vi "2ndStrikerNormalV2.vi"(0 "Início de pass state":bool=TRUE, 4 "Impulso de\ntime elapsed":bool=TRUE, 5 "Force Start":bool, 6 "atacando ao contrário?":bool=TRUE, 7 "AI Parameters":T1={"GotoKick"={"Dist do cone a frente"=150.0, "attacker farback"=1500.0, "Perto"=300.0, "min dist to kick"=150.0, "kick eps"=0.0, "Time to transition"=0.05}, "Attacker"={"CC chute"=0.09, "CC passe"=0.045, "Kick Force"=100.0, "ball-robot Kick"=200.0, "ball-robot Pass"=0.3, "drible\nAttk"=FALSE}, "Defender"={"D max"=1700.0, "Vel p/ robô av"=1000.0, "Kick Force"=100.0, "D atk-def"=0.0, "D farback"=0.0, "drible\ndef"=FALSE, "drible\ngoalie"=FALSE}, "Timeout"={"Field/v in x"=6.0, "Dist Robots"=300, "Dist up in y"=300}, "Pose Striker"={"dist"=200.0, "Numeric"=-4.0, "dist 2"=200.0, "drible\nstriker"=FALSE}, "Dist Stop"=300.0, "D ball out"=200, "D central gap "=150.0, "T pass"=0.0, "Force ++"=0.0, "range kick"=0.0, "Chute alto"=TRUE, "Marcador novo"=TRUE, "drible"=FALSE, "D drible"=300.0, "Versão Striker"=enum."3", "Defesa"=enum."ManMark", "Marcador"=enum."Marcar Segundo mais perigoso", "Receptor passe"=enum."2nd Striker", "Área"=enum."Quadrada"} {"D drible" format="%#_13g"; "D central gap" format="%#_13g"; "Dist Stop" format="%#_13g"; "Pose Striker"."Numeric" format="%#_13g"; "Defender"."Kick Force" format="%#_13g"; "Defender"."Vel p/ robô av" format="%#_13g"; "Attacker"."ball-robot Kick" format="%#_13g"; "Attacker"."Kick Force" format="%#_13g"; "Attacker"."CC passe" format="%#_13g"; "Attacker"."CC chute" format="%#_13g"; "GotoKick"."kick eps" format="%#_13g"; "GotoKick"."min dist to kick" format="%#_13g"; "GotoKick"."Perto" format="%#_13g"; "GotoKick"."attacker farback" format="%#_13g"; "GotoKick"."Dist do cone a frente" format="%#_13g"}, 8 "IA Input":T9={"our_robots"=[], "enemy_robots"=[], "balls"=[], "geometry"={"line_width"=0, "field_length"=0, "field_width"=0, "boundary_width"=0, "referee_width"=0, "goal_width"=0, "goal_depth"=0, "goal_wall_width"=0, "center_circle_radius"=0, "defense_radius"=0, "defense_stretch"=0, "free_kick_from_defense_dist"=0, "penalty_spot_from_field_line_dist"=0, "penalty_line_from_spot_dist"=0}, "IA Judge"={"stage"="", "command"="", "our_goalie_id"=0.0, "enemy_goalie_id"=0.0, "command enum"=enum."Halt", "Time"=enum."Azul"}, "Received Timestamp"=timestamp(0 s since 1904-01-01), "Events"={"Touch"=FALSE, "Ball out"=FALSE, "id touch"=0.0, "Ball out of \nVision"=FALSE, "Ball inside \nGoalie area"=FALSE, "Robot not responding"=FALSE, "Robots responding status"=[1.0, 1.0, 1.0, 1.0, 1.0, 1.0], "Enemy Ball \nPossession"=FALSE, "Pass State"=FALSE, "id end of pass"=0.0, "Kick"=FALSE, "Id ini Possession"=0.0, "Ball Possesion"=FALSE, "Id Possesion"=0.0, "Direct Kick"=FALSE, "2nd Strk Ativo"=FALSE}}, 9 "balls":T7[](array[typedef])=[{"x"=-2165.869384765625, "y"=510.4085693359375, "timestamp"=timestamp(2082758857.4639893 s since 1904-01-01), "Vel_x"=0.0, "Vel_y"=0.0, "Pos Bola Est"=[]}], 10 "Field Size in":T8={"line_width"=10, "field_length"=6000, "field_width"=4000, "boundary_width"=250, "referee_width"=425, "goal_width"=700, "goal_depth"=180, "goal_wall_width"=20, "center_circle_radius"=500, "defense_radius"=500, "defense_stretch"=350, "free_kick_from_defense_dist"=700, "penalty_spot_from_field_line_dist"=450, "penalty_line_from_spot_dist"=350}, 11 "Robot in":T2={"id"=5, "function"=enum."Attacker", "x"=-1842.5054931640625, "y"=520.60986328125, "orientation"=-2.7555055618286133, "v_tangent"=0.0, "v_normal"=0.0, "v_ang"=0.0, "kick_x"=0.0, "kick_z"=0.0, "dribble"=FALSE, "Timestamp"=timestamp(2082758857.4639893 s since 1904-01-01), "estimatives"={"est_v_tangent"=0.0, "est_v_normal"=0.0, "est_vx"=0.0, "est_vy"=0.0, "Pos Robot Est"=[]}, "dest_x_kick"=0.0, "dest_y_kick"=0.0, "Gap Coord"=[], "States"=enum."GoToTangent", "Path "=[], "Path  Smooth"=[], "Dest"=[]}) -> (2 "Robot out":T2={"id"=5, "function"=enum."Attacker", "x"=-1842.5054931640625, "y"=520.60986328125, "orientation"=-2.7555055618286133, "v_tangent"=-0.08361641967936218, "v_normal"=-0.20513016702014014, "v_ang"=0.24456003022714357, "kick_x"=0.0, "kick_z"=0.0, "dribble"=FALSE, "Timestamp"=timestamp(2082758857.4639893 s since 1904-01-01), "estimatives"={"est_v_tangent"=0.0, "est_v_normal"=0.0, "est_vx"=0.0, "est_vy"=0.0, "Pos Robot Est"=[]}, "dest_x_kick"=0.0, "dest_y_kick"=0.0, "Gap Coord"=[], "States"=enum."GoToTangent", "Path "=[], "Path  Smooth"=[], "Dest"=[]})   [LabVIEW 2017]
uses:
  Core/AI Robot.ctl
  Functions Enum.ctl
  AttackerStates.ctl
  Path Planning/RRT/PathDests.ctl
  Path Planning/RRT/PathDest.ctl
  Core/AI Input.ctl
  Core/AI Ball.ctl
  Core/Field Size.ctl
  Core/AI Judge.ctl
  Command Enum.ctl
  Util/Events/Events.ctl
  AI Parameters.ctl
panel:
  in  "Wait pass perpendicular?":bool=TRUE
  in  "Marcador sempre":bool
  out "size(s)":i32
  in  "IDattacker":dbl
  in  "Yattacker":dbl
  in  "Xattacker":dbl
  out "States":T4
  out "sentido":dbl
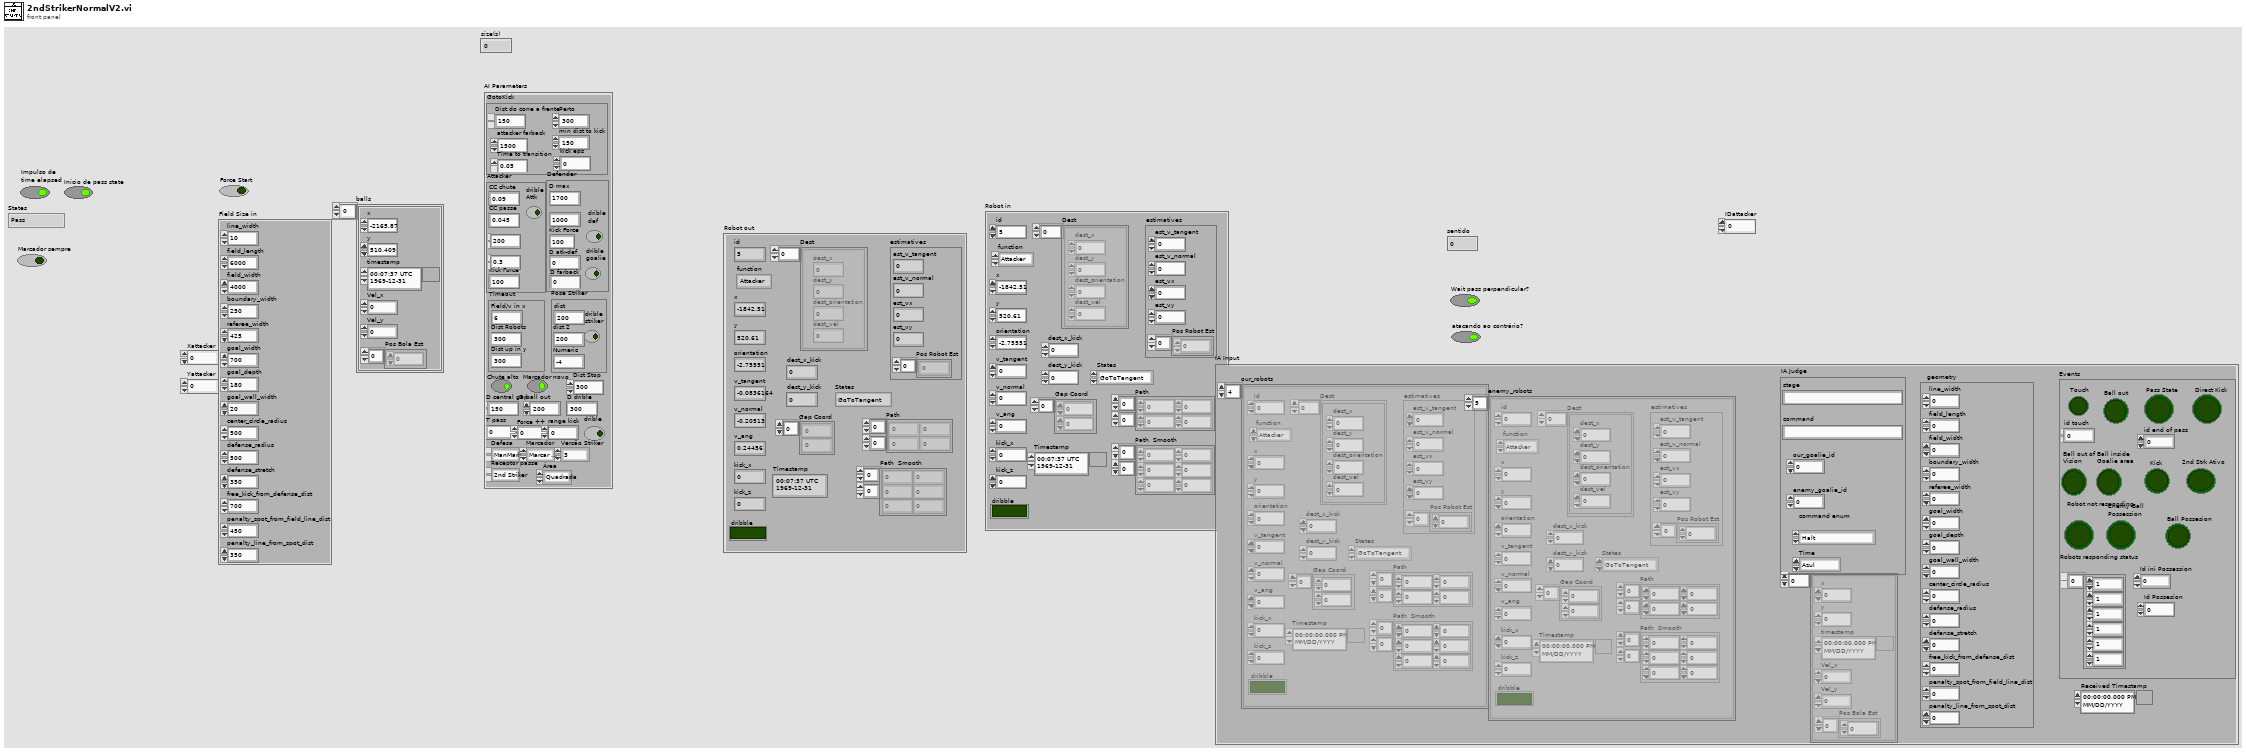
[diagram p1: front panel]
types:
  T1 = typedef "AI Parameters.ctl" = cluster{"GotoKick":cluster{"Dist do cone a frente":dbl, "attacker farback":dbl, "Perto":dbl, "min dist to kick":dbl, "kick eps":dbl, "Time to transition":dbl}, "Attacker":cluster{"CC chute":dbl, "CC passe":dbl, "Kick Force":dbl, "ball-robot Kick":dbl, "ball-robot Pass":dbl, "drible\nAttk":bool}, "Defender":cluster{"D max":dbl, "Vel p/ robô av":dbl, "Kick Force":dbl, "D atk-def":dbl, "D farback":dbl, "drible\ndef":bool, "drible\ngoalie":bool}, "Timeout":cluster{"Field/v in x":dbl, "Dist Robots":u32, "Dist up in y":u32}, "Pose Striker":cluster{"dist":dbl, "Numeric":dbl, "dist 2":dbl, "drible\nstriker":bool}, "Dist Stop":dbl, "D ball out":i32, "D central gap ":dbl, "T pass":dbl, "Force ++":dbl, "range kick":dbl, "Chute alto":bool, "Marcador novo":bool, "drible":bool, "D drible":dbl, "Versão Striker":enum16{"Auto", "3", "2", "1"}, "Defesa":enum16{"ManMark", "Barreira"}, "Marcador":enum16{"Marcar Segundo mais perigoso", "Marcar o mais perigoso"}, "Receptor passe":enum16{"Auto", "2nd Striker", "Striker"}, "Área":enum16{"Quadrada", "Circular"}}
  T2 = typedef "AI Robot.ctl" = cluster{"id":u32, "function":T3, "x":dbl, "y":dbl, "orientation":dbl, "v_tangent":dbl, "v_normal":dbl, "v_ang":dbl, "kick_x":dbl, "kick_z":dbl, "dribble":bool, "Timestamp":timestamp, "estimatives":cluster{"est_v_tangent":dbl, "est_v_normal":dbl, "est_vx":dbl, "est_vy":dbl, "Pos Robot Est":dbl[]}, "dest_x_kick":dbl, "dest_y_kick":dbl, "Gap Coord":dbl[], "States":T4, "Path ":dbl[][], "Path  Smooth":dbl[][], "Dest":T5}
  T3 = typedef "Functions Enum.ctl" = enum16{"2nd Striker", "Attacker", "Goalie", "Defender", "Striker", "Goto 0", "Dummy", "Kicker", "ZigZag 0", "ZigZag 1", "ZigZag 2", "ZigZag 3", "ZigZag 4", "ZigZag 5", "ZigZag 6", "ZigZag 7", "ZigZag 8", ""}
  T4 = typedef "AttackerStates.ctl" = enum16{"Pass", "GoToTangent", "BallGetting", "GoToKick", ""}
  T5 = typedef "PathDests.ctl" = T6[]
  T6 = typedef "PathDest.ctl" = cluster{"dest_x":dbl, "dest_y":dbl, "dest_orientation":dbl, "dest_vel":dbl}
  T7 = typedef "AI Ball.ctl" = cluster{"x":dbl, "y":dbl, "timestamp":timestamp, "Vel_x":dbl, "Vel_y":dbl, "Pos Bola Est":dbl[]}
  T8 = typedef "Field Size.ctl" = cluster{"line_width":u32, "field_length":u32, "field_width":u32, "boundary_width":u32, "referee_width":u32, "goal_width":u32, "goal_depth":u32, "goal_wall_width":u32, "center_circle_radius":u32, "defense_radius":u32, "defense_stretch":u32, "free_kick_from_defense_dist":u32, "penalty_spot_from_field_line_dist":u32, "penalty_line_from_spot_dist":u32}
  T9 = typedef "AI Input.ctl" = cluster{"our_robots":T2[], "enemy_robots":T2[], "balls":T7[], "geometry":T8, "IA Judge":T10, "Received Timestamp":timestamp, "Events":T12}
  T10 = typedef "AI Judge.ctl" = cluster{"stage":string, "command":string, "our_goalie_id":dbl, "enemy_goalie_id":dbl, "command enum":T11, "Time":enum16{"Azul", "Amarelo"}}
  T11 = typedef "Command Enum.ctl" = enum16{"Halt", "Stop", "Force Start", "PKA Normal Start", "Prepare Kickoff Ally", "PKE Normal Start", "Prepare Kickoff Enemy", "Prepare Penalty Ally", "PPA Normal Start", "Prepare Penalty Enemy", "PPE Normal Start", "Direct Free Enemy", "Direct Free Ally", "Indirect Free Enemy", "Indirect Free Ally", "Timeout Enemy", "Timeout Ally", "Goal Enemy", "Goal Ally", "Ball Placement Enemy", "Ball Placement Ally", "Normal Half Time", "Extra Time Break", "Extra Half Time", "None", "Post Game"}
  T12 = typedef "Events.ctl" = cluster{"Touch":bool, "Ball out":bool, "id touch":dbl, "Ball out of \nVision":bool, "Ball inside \nGoalie area":bool, "Robot not responding":bool, "Robots responding status":dbl[], "Enemy Ball \nPossession":bool, "Pass State":bool, "id end of pass":dbl, "Kick":bool, "Id ini Possession":dbl, "Ball Possesion":bool, "Id Possesion":dbl, "Direct Kick":bool, "2nd Strk Ativo":bool}
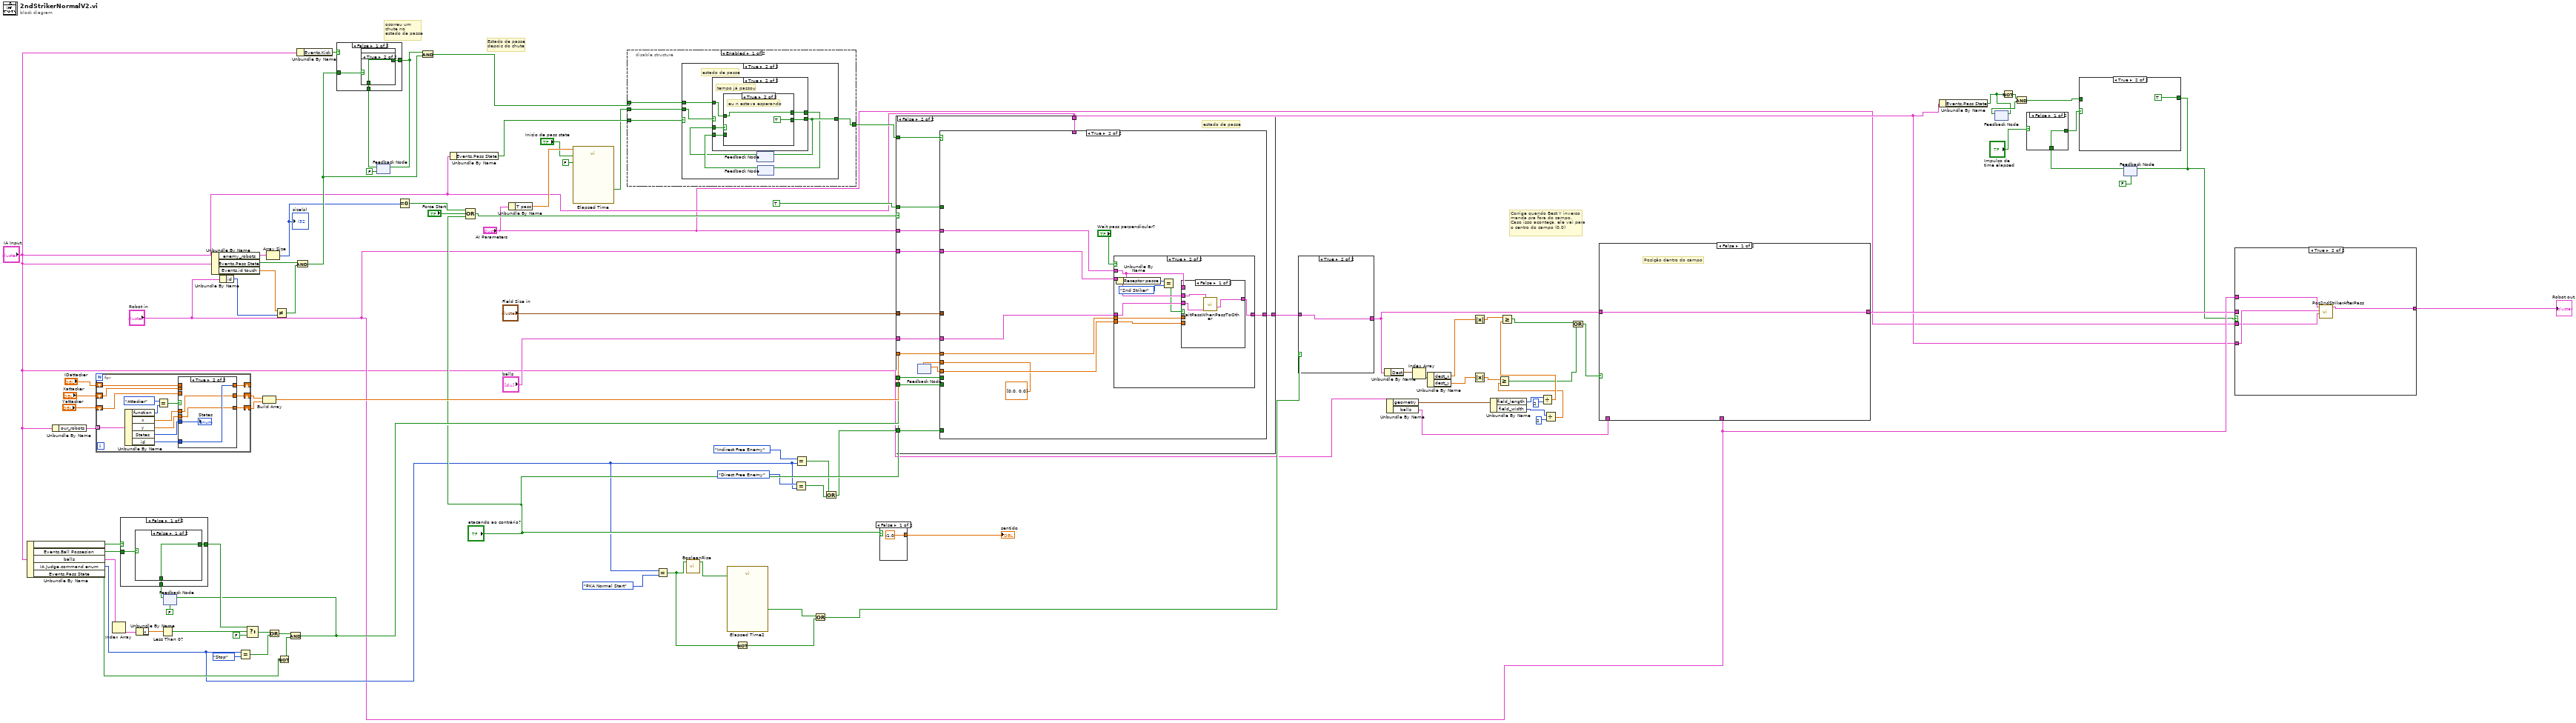
[diagram p0: block diagram]
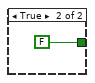
[diagram p2: hidden frame]
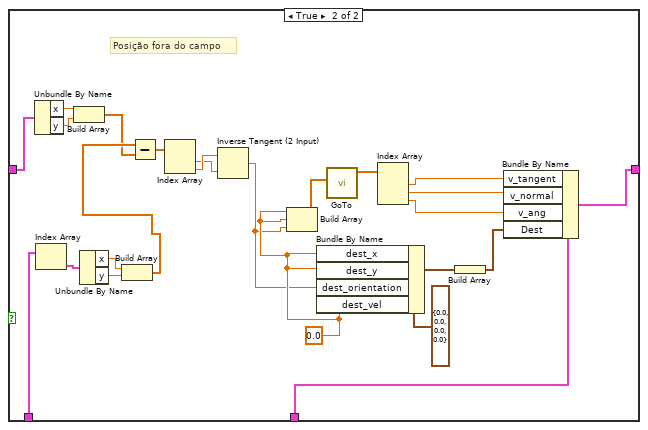
[diagram p5: hidden frame]
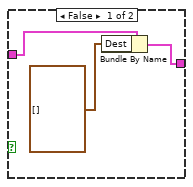
[diagram p6: hidden frame]
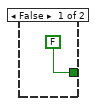
[diagram p7: hidden frame]
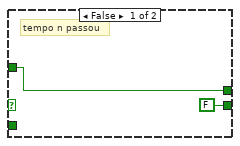
[diagram p8: hidden frame]
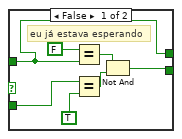
[diagram p9: hidden frame]
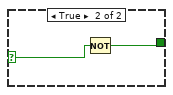
[diagram p11: hidden frame]
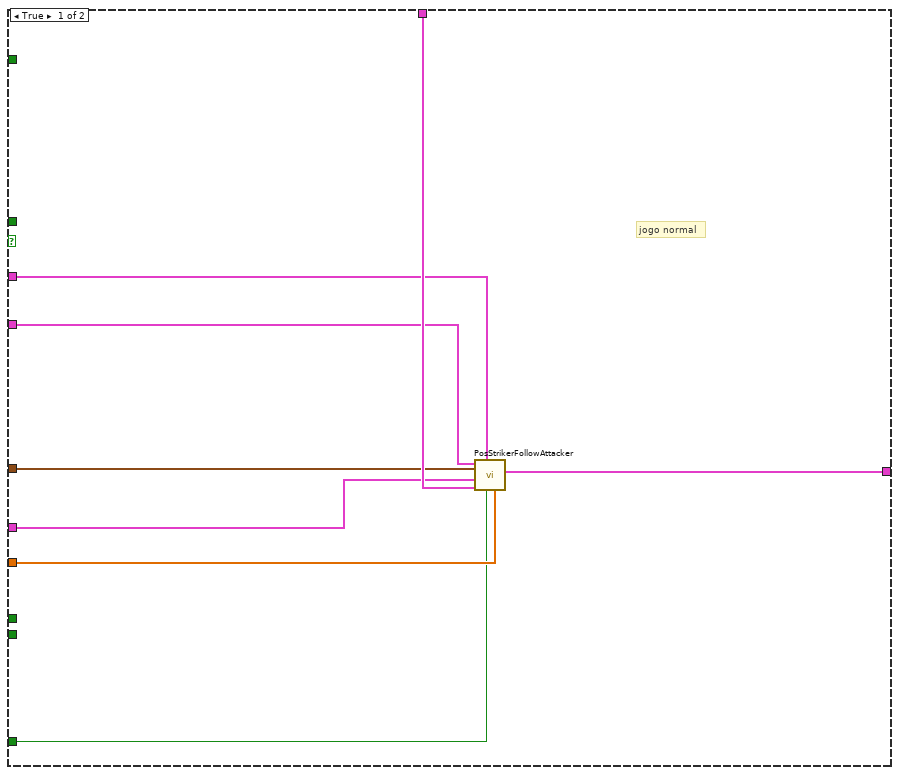
[diagram p13: hidden frame]
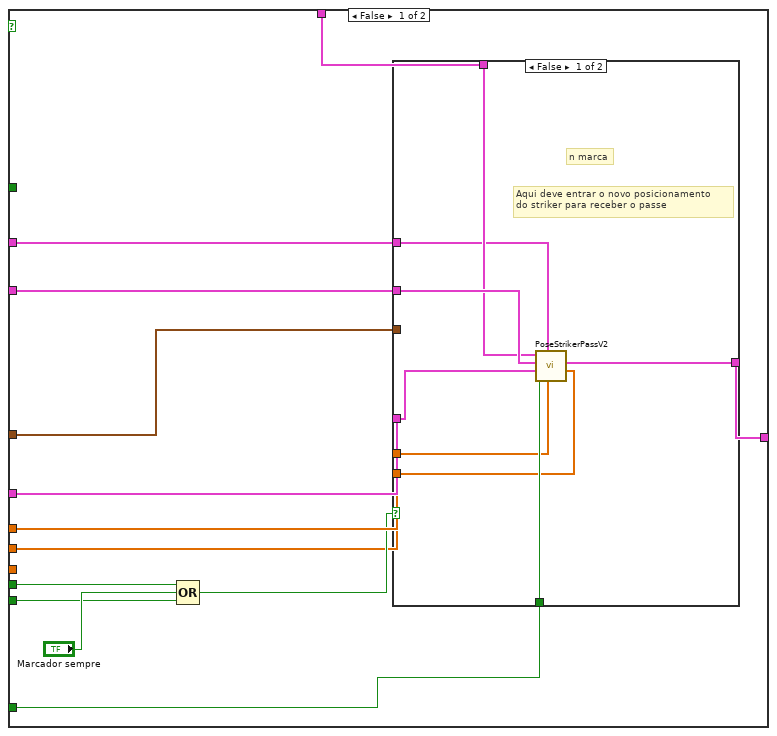
[diagram p14: hidden frame]
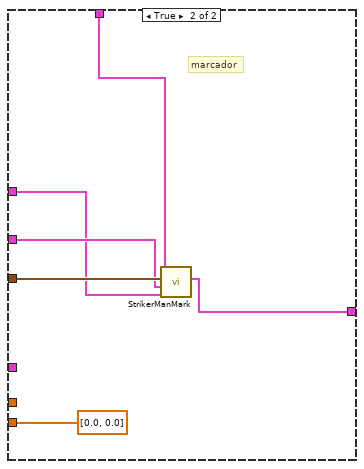
[diagram p15: hidden frame]
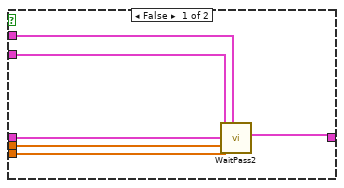
[diagram p16: hidden frame]
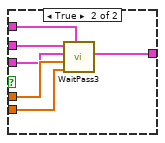
[diagram p17: hidden frame]
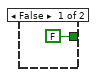
[diagram p19: hidden frame]
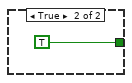
[diagram p20: hidden frame]
diagram:
  # "Corrige quando Best Y inverso\nmanda pra fora do campo.\nCaso isso aconteça, ele vai para\no centro do campo (0,0)"
  # "ocorreu um \nchute no\nestado de passe"
  # "Estado de passe\ndepois do chute"
  n1 = Unbundle By Name("IA Input") -> ("Events.Enemy Ball \nPossession"=w74:bool, "Events.Ball Possesion"=w73:bool, "balls"=w71:T7[], "IA Judge.command enum"=w42:T11, "Events.Pass State"=w61:bool)
  n2 = Unbundle By Name("IA Input") -> ("our_robots"=w89:T2[])
  n3 = for {
    tunnel: w89 -> [w104] mode=indexing
    shift-right: [w100] -> w85
    shift-left: "Xattacker" -> [w98]
    shift-right: [w99] -> w84
    shift-left: "Yattacker" -> [w97]
    shift-right: [w101] -> _
    shift-left: "IDattacker" -> [w96]
    n4 = Unbundle By Name(w104) -> ("function"=w109:T3, "x"=w106:dbl, "y"=w105:dbl, "States"=w103:T4, "id"=w102:u32)
    n5 = Equal?(x=Functions_Enum."Attacker", y=w109) -> (x = y?=w107:bool)
    n6 = case shown="True" w107 {
      tunnel: w106 -> [_ w114]
      tunnel: w105 -> [_ w113]
      tunnel: w103 -> [_ w116]
      tunnel: w102 -> [_ w115]
      tunnel: [w110 w115] -> w101
      tunnel: [w112 w114] -> w100
      tunnel: [w111 w113] -> w99
      tunnel: w98 -> [w112 _]
      tunnel: w97 -> [w111 _]
      tunnel: w96 -> [w110 _]
      frame False {
      }
      frame True {
        "States" <- w116
      }
    }
  }
  n7 = Index Array(array=w71) -> (element=w70:T7)  [unwired: 1 in]
  n8 = Unbundle By Name(w70) -> ("x"=w69:dbl)
  n9 = Less Than 0?(x=w69) -> (x < 0?=w68:bool)
  n10 = feedback #1(FALSE) -> (w72:bool)
  n11 = case shown="False" w74 {
    selector: w74 -> [_ w123]
    tunnel: [w118 w123] -> w67
    tunnel: w73 -> [w119 _]
    tunnel: w72 -> [w117 _]
    frame False {
      n12 = case shown="False" w119 {
        selector: w119 -> [_ w121]
        tunnel: [w120 w122] -> w118
        tunnel: w117 -> [w120 _]
        frame False {
        }
        frame True {
          n13 = Not(x=w121) -> (.not. x?=w122:bool)
        }
      }
    }
    frame True {
    }
  }
  n14 = Unbundle By Name("IA Input") -> ("enemy_robots"=w54:T2[], "Events.Pass State"=w90:bool, "Events.id touch"=w79:dbl)
  n15 = Unbundle By Name("Robot in") -> ("id"=w78:u32)
  n16 = Equal?(x=w42, y=Command_Enum."Stop") -> (x = y?=w64:bool)
  n17 = Select(t=w67, s=w68, f=FALSE) -> (s? t:f=w65:bool)
  n18 = Build Array(w85, w84) -> (w83:dbl[])
  n19 = Array Size(array=w54) -> (size(s)=w52:i32)
  "size(s)" <- w52
  n20 = Or(x=w65, y=w64) -> (x .or. y?=w62:bool)
  n21 = Not Equal?(x=w79, y=w78) -> (x != y?=w80:bool)
  n22 = Not(x=w61) -> (.not. x?=w60:bool)
  n23 = And(x=w62, y=w60) -> (x .and. y?=w59:bool)
  n24 = feedback-in #1(w59) -> ()
  n25 = Unbundle By Name("IA Input") -> ("Events.Kick"=w94:bool)
  n26 = Compound Arithmetic op=AND(w90, w80) -> (w81:bool)
  n27 = feedback #2(FALSE) -> (w92:bool)
  n28 = case shown="False" w94 {
    tunnel: [w125 TRUE] -> w93
    tunnel: w92 -> [w124 _]
    tunnel: w81 -> [w126 _]
    frame False {
      n29 = case shown="True" w126 {
        tunnel: [FALSE w128] -> w125
        tunnel: w124 -> [_ w128]
        frame False {
        }
        frame True {
        }
      }
    }
    frame True {
    }
  }
  n30 = feedback-in #2(w93) -> ()
  n31 = Equal To 0?(x=w52) -> (x = 0?=w53:bool)
  n32 = And(x=w93, y=w81) -> (x .and. y?=w57:bool)
  n33 = Unbundle By Name("IA Input") -> ("Events.Pass State"=w56:bool)
  n34 = Compound Arithmetic op=OR(w53, "Force Start", "atacando ao contrário?") -> (w50:bool)
  n35 = Unbundle By Name("AI Parameters") -> ("T pass"=w51:dbl)
  n36 = call "Elapsed Time"("Time Target (s)"=w51, "Reset"="Início de pass state", "Auto Reset"=FALSE) -> ("Time has Elapsed"=w55:bool)  [unwired: 9 in, 7 out]
  n37 = disable-structure shown="Enabled" {
    disable-tunnel: w55 -> [w131 _]
    disable-tunnel: [w133 w157] -> w58
    disable-tunnel: w57 -> [w132 w157]
    disable-tunnel: w56 -> [w130 _]
    frame Enabled {
      n38 = case shown="True" w130 {
        tunnel: [FALSE w140] -> w133
        tunnel: w132 -> [_ w139]
        tunnel: w131 -> [_ w136]
        frame False {
        }
        frame True {
          # "estado de passe"
          n39 = feedback #3() -> (w135:bool)  [unwired: 1 in]
          n40 = feedback #4() -> (w137:bool)  [unwired: 1 in]
          n41 = case shown="True" w136 {
            tunnel: [FALSE w146] -> w140
            tunnel: w139 -> [w141 w145]
            tunnel: [w141 w143] -> w138
            tunnel: w137 -> [_ w144]
            tunnel: w135 -> [_ w147]
            frame False {
              # "tempo n passou"
            }
            frame True {
              # "tempo já passou"
              n42 = case shown="True" w147 {
                tunnel: [w149 TRUE] -> w146
                tunnel: w145 -> [w148 w155]
                tunnel: w144 -> [w150 _]
                tunnel: [w148 w155] -> w143
                frame False {
                  # "eu já estava esperando"
                  n43 = Equal?(x=FALSE, y=w148) -> (x = y?=w151:bool)
                  n44 = Equal?(x=w150, y=TRUE) -> (x = y?=w152:bool)
                  n45 = Not And(1:w152, 2:w151) -> (0:w149:bool)
                }
                frame True {
                  # "eu n estava esperando"
                }
              }
            }
          }
          n46 = feedback-in #3(w140) -> ()
          n47 = feedback-in #4(w138) -> ()
        }
      }
    }
    frame Disabled {
    }
  }
  n48 = Equal?(x=w42, y=Command_Enum."PKA Normal Start") -> (x = y?=w38:bool)
  n49 = call "BooleanRise.vi"("Test Mode On"=w38) -> ("Boolean"=w40:bool)  [unwired: 10 in]
  n50 = call "Elapsed Time2"("Reset"=w40) -> ("Time has Elapsed"=w36:bool)  [unwired: 11 in, 7 out]
  n51 = Not(x=w38) -> (.not. x?=w37:bool)
  n52 = Equal?(x=Command_Enum."Direct Free Enemy", y=w42) -> (x = y?=w45:bool)
  n53 = Equal?(x=Command_Enum."Indirect Free Enemy", y=w42) -> (x = y?=w44:bool)
  n54 = Or(x=w36, y=w37) -> (x .or. y?=w35:bool)
  n55 = Compound Arithmetic op=OR(w44, w45) -> (w43:bool)
  n56 = case shown="False" "atacando ao contrário?" {
    tunnel: [-1.0 1.0] -> w95
    frame False {
    }
    frame True {
    }
  }
  "sentido" <- w95
  n57 = case shown="False" w50 {
    tunnel: w58 -> [_ w173]
    tunnel: TRUE -> [_ w174]
    tunnel: "Robot in" -> [w166 w181]
    tunnel: w83 -> [w163 w180]
    tunnel: "atacando ao contrário?" -> [w162 w179]
    tunnel: "Field Size in" -> [w165 w178]
    tunnel: "balls" -> [w164 w177]
    tunnel: "IA Input" -> [w167 w176]
    tunnel: [w161 w175] -> w39
    tunnel: "AI Parameters" -> [w160 w172]
    tunnel: w59 -> [_ w171]
    tunnel: w43 -> [_ w168]
    frame True {
      # "jogo normal"
      n58 = call "PosStrikerFollowAttacker.vi"("Pos Attacker"=w163, "atacando ao contrário?"=w162, "AI Parameters"=w160, "IA Input"=w167, "balls"=w164, "Field Size in"=w165, "Robot in"=w166) -> ("Robot out"=w161:T2)  [unwired: 4 in]
    }
    frame False {
      # "estado de passe"
      n59 = feedback #5() -> (w169:dbl[])  [unwired: 1 in]
      n60 = case shown="True" w173 {
        tunnel: w174 -> [_ _]
        tunnel: w181 -> [w193 w216]
        tunnel: w180 -> [w188 w215]
        tunnel: [w190 w214] -> w175
        tunnel: w179 -> [w194 _]
        tunnel: w178 -> [w187 _]
        tunnel: w177 -> [w192 w213]
        tunnel: w176 -> [w191 _]
        tunnel: w172 -> [w189 w209]
        tunnel: w171 -> [w186 _]
        tunnel: [w183 dbl[] [0.0, 0.0] ("FinalPosition")] -> w170
        tunnel: w169 -> [_ w212]
        tunnel: w168 -> [w182 _]
        frame False {
          n61 = Compound Arithmetic op=OR(w186, "Marcador sempre", w182) -> (w185:bool)
          n62 = case shown="False" w185 {
            tunnel: w194 -> [w202 _]
            tunnel: w193 -> [w201 w207]
            tunnel: w192 -> [w200 _]
            tunnel: w191 -> [w199 w205]
            tunnel: [w198 w206] -> w190
            tunnel: w189 -> [w197 w204]
            tunnel: w188 -> [w196 _]
            tunnel: w187 -> [_ w208]
            tunnel: [w195 dbl[] [0.0, 0.0] ("FinalPosition")] -> w183
            frame False {
              # "n marca"
              # "Aqui deve entrar o novo posicionamento\ndo striker para receber o passe"
              n63 = call "PoseStrikerPassV2.vi"("Array"=w196, "AI Parameters"=w197, "atacando ao contrário?"=w202, "balls"=w200, "Robot in"=w201, "IA Input"=w199) -> ("FinalPosition"=w195:dbl[], "Robot out"=w198:T2)  [unwired: 4 in]
            }
            frame True {
              # "marcador"
              n64 = call "StrikerManMark.vi"("AI Parameters"=w204, "Robot in"=w207, "Field Size in"=w208, "IA Input"=w205) -> ("Robot out"=w206:T2)  [unwired: 6 in, 1 out]
            }
          }
        }
        frame True {
          n65 = case shown="True" "Wait pass perpendicular?" {
            tunnel: w216 -> [w221 w231]
            tunnel: w215 -> [w219 w230]
            tunnel: [w222 w229] -> w214
            tunnel: w213 -> [w220 w228]
            tunnel: w212 -> [w218 w227]
            tunnel: w209 -> [w217 w226]
            frame False {
              n66 = call "WaitPass2.vi"("AI Parameters"=w217, "Best Y Inverso"=w218, "Target"=w219, "balls"=w220, "Robot in"=w221) -> ("Robot out"=w222:T2)  [unwired: 6 in]
            }
            frame True {
              n67 = Unbundle By Name(w226) -> ("Receptor passe"=w225:enum16{"Auto", "2nd Striker", "Striker"})
              n68 = Equal?(x=w225, y=enum16{"Auto", "2nd Striker", "Striker"}."2nd Striker") -> (x = y?=w224:bool)
              n69 = case shown="False" w224 {
                tunnel: w231 -> [w233 w240]
                tunnel: w230 -> [_ w239]
                tunnel: [w234 w238] -> w229
                tunnel: w228 -> [w232 w237]
                tunnel: w227 -> [_ w236]
                tunnel: w226 -> [_ w235]
                frame False {
                  n70 = call "WaitPassWhenPassToOther.vi"("balls"=w232, "Robot in"=w233) -> ("Robot out"=w234:T2)  [unwired: 9 in]
                }
                frame True {
                  n71 = call "WaitPass3.vi"("AI Parameters"=w235, "Best Y Inverso"=w236, "Target"=w239, "balls"=w237, "Robot in"=w240) -> ("Robot out"=w238:T2)  [unwired: 6 in]
                }
              }
            }
          }
        }
      }
      n72 = feedback-in #5(w170) -> ()
    }
  }
  n73 = case shown="True" w35 {
    tunnel: [w242 w244] -> w18
    tunnel: w39 -> [w243 w244]
    frame False {
      n74 = Bundle By Name(cluster=w243, "Dest"=T5 []) -> (w242:T2)
    }
    frame True {
    }
  }
  n75 = Unbundle By Name(w18) -> ("Dest"=w22:T5)
  n76 = Unbundle By Name("IA Input") -> ("geometry"=w34:T8, "balls"=w15:T7[])
  n77 = Index Array(array=w22) -> (element=w21:T6)  [unwired: 1 in]
  n78 = Unbundle By Name(w21) -> ("dest_x"=w20:dbl, "dest_y"=w19:dbl)
  n79 = Absolute Value(x=w20) -> (abs(x)=w29:dbl)
  n80 = Absolute Value(x=w19) -> (abs(x)=w27:dbl)
  n81 = Unbundle By Name(w34) -> ("field_length"=w33:u32, "field_width"=w30:u32)
  n82 = Divide(x=w33, y=2) -> (x/y=w28:dbl)
  n83 = Greater Or Equal?(x=w29, y=w28) -> (x >= y?=w25:bool)
  n84 = Divide(x=w30, y=u32 2) -> (x/y=w26:dbl)
  n85 = Greater Or Equal?(x=w27, y=w26) -> (x >= y?=w24:bool)
  n86 = Or(x=w25, y=w24) -> (x .or. y?=w23:bool)
  n87 = case shown="False" w23 {
    tunnel: [w245 w266] -> w16
    tunnel: w18 -> [w245 w247]
    tunnel: "Robot in" -> [_ w265]
    tunnel: w15 -> [_ w248]
    frame False {
      # "Posição dentro do campo"
    }
    frame True {
      w259 = 0.0 ("dest_vel")
      # "Posição fora do campo"
      n88 = Unbundle By Name(w247) -> ("x"=w255:dbl, "y"=w254:dbl)
      n89 = Index Array(array=w248) -> (element=w258:T7)  [unwired: 1 in]
      n90 = Build Array(w255, w254) -> (w251:dbl[])
      n91 = Unbundle By Name(w258) -> ("x"=w257:dbl, "y"=w256:dbl)
      n92 = Build Array(w257, w256) -> (w252:dbl[])
      n93 = Subtract(x=w252, y=w251) -> (x-y=w253:dbl[])
      n94 = Index Array(array=w253) -> (element #1=w249:dbl, element #2=w250:dbl)  [unwired: 2 in]
      n95 = Inverse Tangent (2 Input)(1:w249, 2:w250) -> (0:w246:dbl)
      n96 = Build Array(w259, w259, w246) -> (w260:dbl[])
      n97 = Bundle By Name(cluster=T6 {"dest_x"=0.0, "dest_y"=0.0, "dest_orientation"=0.0, "dest_vel"=0.0} ("Dest"), "dest_x"=w259, "dest_y"=w259, "dest_orientation"=w246, "dest_vel"=w259) -> (w268:T6)
      n98 = call "GoTo.vi"("Target"=w260) -> ("Output\nVelocity"=w264:dbl[])  [unwired: 9 in, 1 out]
      n99 = Index Array(array=w264) -> (element #1=w263:dbl, element #2=w261:dbl, element #3=w262:dbl)  [unwired: 3 in]
      n100 = Build Array(w268) -> (w267:T6[])
      n101 = Bundle By Name(cluster=w265, "v_tangent"=w263, "v_normal"=w261, "v_ang"=w262, "Dest"=w267) -> (w266:T2)
    }
  }
  n102 = Unbundle By Name("IA Input") -> ("Events.Pass State"=w5:bool)
  n103 = feedback-in #6(w5) -> ()
  n104 = feedback #6() -> (w12:bool)  [unwired: 1 in]
  n105 = Not(x=w5) -> (.not. x?=w4:bool)
  n106 = And(x=w4, y=w12) -> (x .and. y?=w11:bool)
  n107 = feedback #7(FALSE) -> (w7:bool)
  n108 = case shown="False" "Impulso de\ntime elapsed" {
    tunnel: [w270 FALSE] -> w8
    tunnel: w7 -> [w270 _]
    frame False {
    }
    frame True {
    }
  }
  n109 = case shown="True" w8 {
    tunnel: [w272 TRUE] -> w6
    tunnel: w11 -> [w272 _]
    frame False {
    }
    frame True {
    }
  }
  n110 = feedback-in #7(w6) -> ()
  n111 = case shown="True" w6 {
    tunnel: [w274 w278] -> w17
    tunnel: w16 -> [w274 _]
    tunnel: "IA Input" -> [_ w277]
    tunnel: "Robot in" -> [_ w276]
    tunnel: "AI Parameters" -> [_ w275]
    frame False {
    }
    frame True {
      n112 = call "Pos2ndStrikerAfterPass.vi"("AI Parameters"=w275, "IA Input"=w277, "Robot in"=w276) -> ("Robot out"=w278:T2)  [unwired: 8 in]
    }
  }
  "Robot out" <- w17
